vi "AlliGator Is Selected Channel First Channel.vi"(11 "Selected Channel Name":string) -> (3 "First channel?":bool)   [LabVIEW 2021, in "AlliGator Dual-Channel Datasets.lvlib"]
doc: "Identifies what type of channel is selected (<B>First channel</B> = TRUE: G2 or <B>First channel</B> = FALSE: INT).\n\nIn the case of a single-channel dataset, the output is TRUE."
uses:
  AlliGator Dual-Channel Datasets.lvlib
panel:
  # "see the AlliGator License on the block diagram (Ctrl+E or Window:Show Block Diagram)"
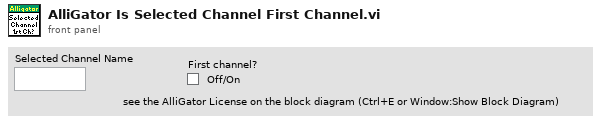
[diagram p1: front panel]
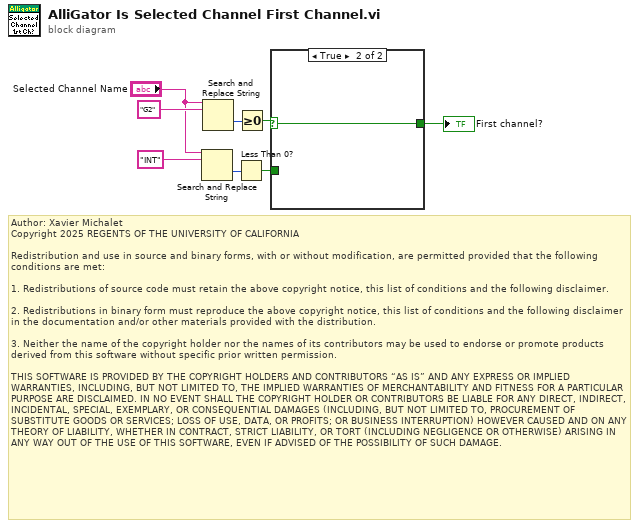
[diagram p0: block diagram]
diagram:
  # "Author: Xavier Michalet\nCopyright 2025 REGENTS OF THE UNIVERSITY OF CALIFORNIA\n\nRedistribution and use in source and binary forms, with or without modification, are permitted provided that the following conditions are met:\n\n1. Redistributions of source code must retain the above copyright notice, this list of conditions and the following disclaimer.\n\n2. Redistributions in binary form must reproduce the above copyright notice, this list of conditions and the following disclaimer in the documentation and/or other materials provided with the distribution.\n\n3. Neither the name of the copyright holder nor the names of its contributors may be used to endorse or promote products derived from this software without specific prior written permission.\n\nTHIS SOFTWARE IS PROVIDED BY THE COPYRIGHT HOLDERS AND CONTRIBUTORS “AS IS” AND ANY EXPRESS OR IMPLIED WARRANTIES, INCLUDING, BUT NOT LIMITED TO, THE IMPLIED WARRANTIES OF MERCHANTABILITY AND FITNESS FOR A PARTICULAR PURPOSE ARE DISCLAIMED. IN NO EVENT SHALL THE COPYRIGHT HOLDER OR CONTRIBUTORS BE LIABLE FOR ANY DIRECT, INDIRECT, INCIDENTAL, SPECIAL, EXEMPLARY, OR CONSEQUENTIAL DAMAGES (INCLUDING, BUT NOT LIMITED TO, PROCUREMENT OF SUBSTITUTE GOODS OR SERVICES; LOSS OF USE, DATA, OR PROFITS; OR BUSINESS INTERRUPTION) HOWEVER CAUSED AND ON ANY THEORY OF LIABILITY, WHETHER IN CONTRACT, STRICT LIABILITY, OR TORT (INCLUDING NEGLIGENCE OR OTHERWISE) ARISING IN ANY WAY OUT OF THE USE OF THIS SOFTWARE, EVEN IF ADVISED OF THE POSSIBILITY OF SUCH DAMAGE."
  n1 = Search and Replace String(input string="Selected Channel Name", search string="INT") -> (offset past replacement=w6:i32)  [unwired: 6 in, 3 out]
  n2 = Search and Replace String(input string="Selected Channel Name", search string="G2" ("substring (\"\")")) -> (offset past replacement=w8:i32)  [unwired: 6 in, 3 out]
  n3 = Less Than 0?(x=w6) -> (x < 0?=w1:bool)
  n4 = Greater Or Equal To 0?(x=w8) -> (x >= 0?=w3:bool)
  n5 = case shown="True" w3 {
    selector: w3 -> [_ w10]
    tunnel: [w9 w10] -> w2
    tunnel: w1 -> [w9 _]
    frame False {
      # "not G2 AND no INT =>single channel"
    }
    frame True {
    }
  }
  "First channel?" <- w2
